vi "Randomized Start Positions.vi"(10 "Player Count":i32, 11 "Size":i32) -> (3 "Positions":T1[](array[typedef]))   [LabVIEW 2020, in "SquareBattle.lvlib" / "Game.lvclass"]
uses:
  Game.lvclass
  Position.ctl
  4bf63a30-6ba3-4053-8b47-148aedb745aa.vi
  SquareBattle.lvlib
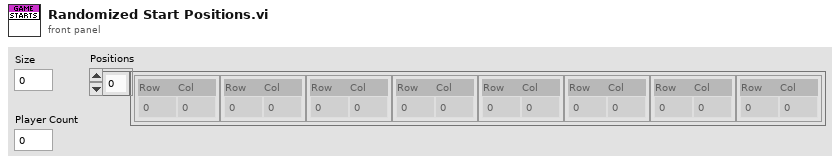
[diagram p1: front panel]
types:
  T1 = typedef "SquareBattle.lvlib/Position.ctl" = cluster{"Row":i32, "Col":i32}
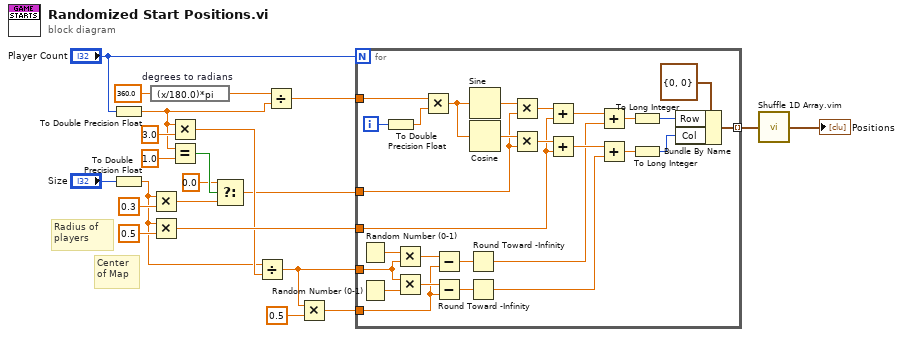
[diagram p0: block diagram]
diagram:
  # "Center of Map"
  # "Radius of players"
  n1 = To Double Precision Float(number="Player Count") -> (double precision float=w7:dbl)
  n2 = To Double Precision Float(number="Size") -> (double precision float=w11:dbl)
  n3 = expression code="(x/180.0)*pi" "degrees to radians"(360.0) -> (w20:dbl)
  n4 = Multiply(x=w11, y=0.3) -> (x*y=w9:dbl)
  n5 = Multiply(x=w11, y=0.5) -> (x*y=w16:dbl)
  n6 = Multiply(x=w7, y=3.0) -> (x*y=w12:dbl)
  n7 = Equal?(x=w7, y=1.0) -> (x = y?=w5:bool)
  n8 = Select(t=0.0, s=w5, f=w9) -> (s? t:f=w8:dbl)
  n9 = Divide(x=w11, y=w12) -> (x/y=w2:dbl)
  n10 = Divide(x=w20, y=w7) -> (x/y=w22:dbl)
  n11 = Multiply(x=w2, y=0.5) -> (x*y=w1:dbl)
  n12 = for {
    N: "Player Count" -> [_]
    tunnel: w22 -> [w49]
    tunnel: w8 -> [w44]
    tunnel: w16 -> [w41]
    tunnel: [w37] -> w15 mode=indexing
    tunnel: w2 -> [w27]
    tunnel: w1 -> [w25]
    i -> [w50]
    n13 = Random Number (0-1)() -> (number: 0 to 1=w32:dbl)
    n14 = Random Number (0-1)() -> (number: 0 to 1=w31:dbl)
    n15 = To Double Precision Float(number=w50) -> (double precision float=w48:dbl)
    n16 = Multiply(x=w32, y=w27) -> (x*y=w28:dbl)
    n17 = Multiply(x=w27, y=w31) -> (x*y=w26:dbl)
    n18 = Multiply(x=w49, y=w48) -> (x*y=w47:dbl)
    n19 = Subtract(x=w28, y=w25) -> (x-y=w23:dbl)
    n20 = Subtract(x=w26, y=w25) -> (x-y=w24:dbl)
    n21 = Round Toward -Infinity(1:w23) -> (0:w30:dbl)
    n22 = Round Toward -Infinity(1:w24) -> (0:w29:dbl)
    n23 = Sine(x=w47) -> (sin(x)=w45:dbl)
    n24 = Cosine(x=w47) -> (cos(x)=w46:dbl)
    n25 = Multiply(x=w45, y=w44) -> (x*y=w42:dbl)
    n26 = Multiply(x=w46, y=w44) -> (x*y=w43:dbl)
    n27 = Add(x=w42, y=w41) -> (x+y=w36:dbl)
    n28 = Add(x=w43, y=w41) -> (x+y=w35:dbl)
    n29 = Add(x=w36, y=w30) -> (x+y=w33:dbl)
    n30 = Add(x=w35, y=w29) -> (x+y=w34:dbl)
    n31 = To Long Integer(number=w33) -> (32bit integer=w39:i32)
    n32 = To Long Integer(number=w34) -> (32bit integer=w38:i32)
    n33 = Bundle By Name(cluster=T1 {"Row"=0, "Col"=0} ("Position"), "Row"=w39, "Col"=w38) -> (w37:T1)
  }
  n34 = call "Shuffle 1D Array.vim"("array"=w15) -> ("shuffled array"=→"Positions":T1[])  [unwired: 4 in]
